vi "Autonomous Independent.vi"   [LabVIEW 2015]
doc: "This VI is called when autonomous begins, and will automatically be terminated when autonomous ends. You can carry out timed or sensor driven robot movement independently without needing to return to the caller."
uses:
  <vilib>/Rock Robotics/WPI/Utilities/WPI_GetSetVariantRefNum.vi
  <vilib>/Rock Robotics/Network Tables/NT Read Number.vi
  <vilib>/Rock Robotics/Network Tables/NT Write Numeric Array.vi
panel:
  # "Be sure to right-click and choose Data Operations>>Make Current Value default if you want to save the array values with the VI"
types:
  T1 = typedef "WPI_JoystickDevRef.ctl" = cluster{"Device":T2}
  T2 = typedef "WPI_JoystickDeviceEnum.ctl" = enum16{"USB 0", "USB 1", "USB 2", "USB 3", "USB 4", "USB 5"}
  T3 = typedef "WPI_EncoderDevRef.ctl" = cluster{"DevStatus":errorcluster, "EncoderIndex":T4, "CounterIndex":T5, "DistancePerCount":dbl, "Decoding Type":T6}
  T4 = typedef "FPGA_EncoderIdx.ctl" = enum8{"Enc 0", "Enc 1", "Enc 2", "Enc 3", "Enc 4", "Enc 5", "Enc 6", "Enc 7", "Invalid"}
  T5 = typedef "FPGA_CounterCtrSystemIndex.ctl" = enum8{"Ctr 0", "Ctr 1", "Ctr 2", "Ctr 3", "Ctr 4", "Ctr 5", "Ctr 6", "Ctr 7", "Invalid"}
  T6 = typedef "WPI_EncoderType.ctl" = enum16{"1x", "2x", "4x"}
  T7 = typedef "WPI_MotorControlDeviceRef.ctl" = cluster{"DeviceStatus":errorcluster, "Type":T8, "PWM":cluster{"PWM Channel":T9, "DeadBand":T10}, "CAN":cluster{"Device Number":u8, "Control Mode":T11, "Semaphore":T12, "Max Vout":dbl, "TalonSRX Control Mode":T13}, "Invert":bool}
  T8 = typedef "WPI_MotorControlType.ctl" = enum16{"PWM", "CAN", "CANTalonSRX"}
  T9 = typedef "FPGA_DIOPWMChannel.ctl" = enum8{"PWM 0", "PWM 1", "PWM 2", "PWM 3", "PWM 4", "PWM 5", "PWM 6", "PWM 7", "PWM 8", "PWM 9", "PWM MXP 0", "PWM MXP 1", "PWM MXP 2", "PWM MXP 3", "PWM MXP 4", "PWM MXP 5", "PWM MXP 6", "PWM MXP 7", "PWM MXP 8", "PWM MXP 9", "Invalid"}
  T10 = typedef "WPI_PWMDeadband.ctl" = cluster{"Name":string, "maxPositivePwm":i32, "minPositivePwm":i32, "centerPwm":i32, "maxNegativePwm":i32, "minNegativePwm":i32, "angularRange":u16}
  T11 = typedef "WPI_CANJaguar_ControlMode.ctl" = enum8{"Percent VBus", "Current", "Speed", "Position", "Voltage"}
  T12 = typedef "Semaphore RefNum" = refnum<k1>
  T13 = typedef "WPI_CANTalonSRX_APIControlMode.ctl" = enum8{"Percent VBus", "Speed", "Position", "Slave", "Unchanged / Invalid", "Voltage Compensation", "Current", "Motion Profile"}
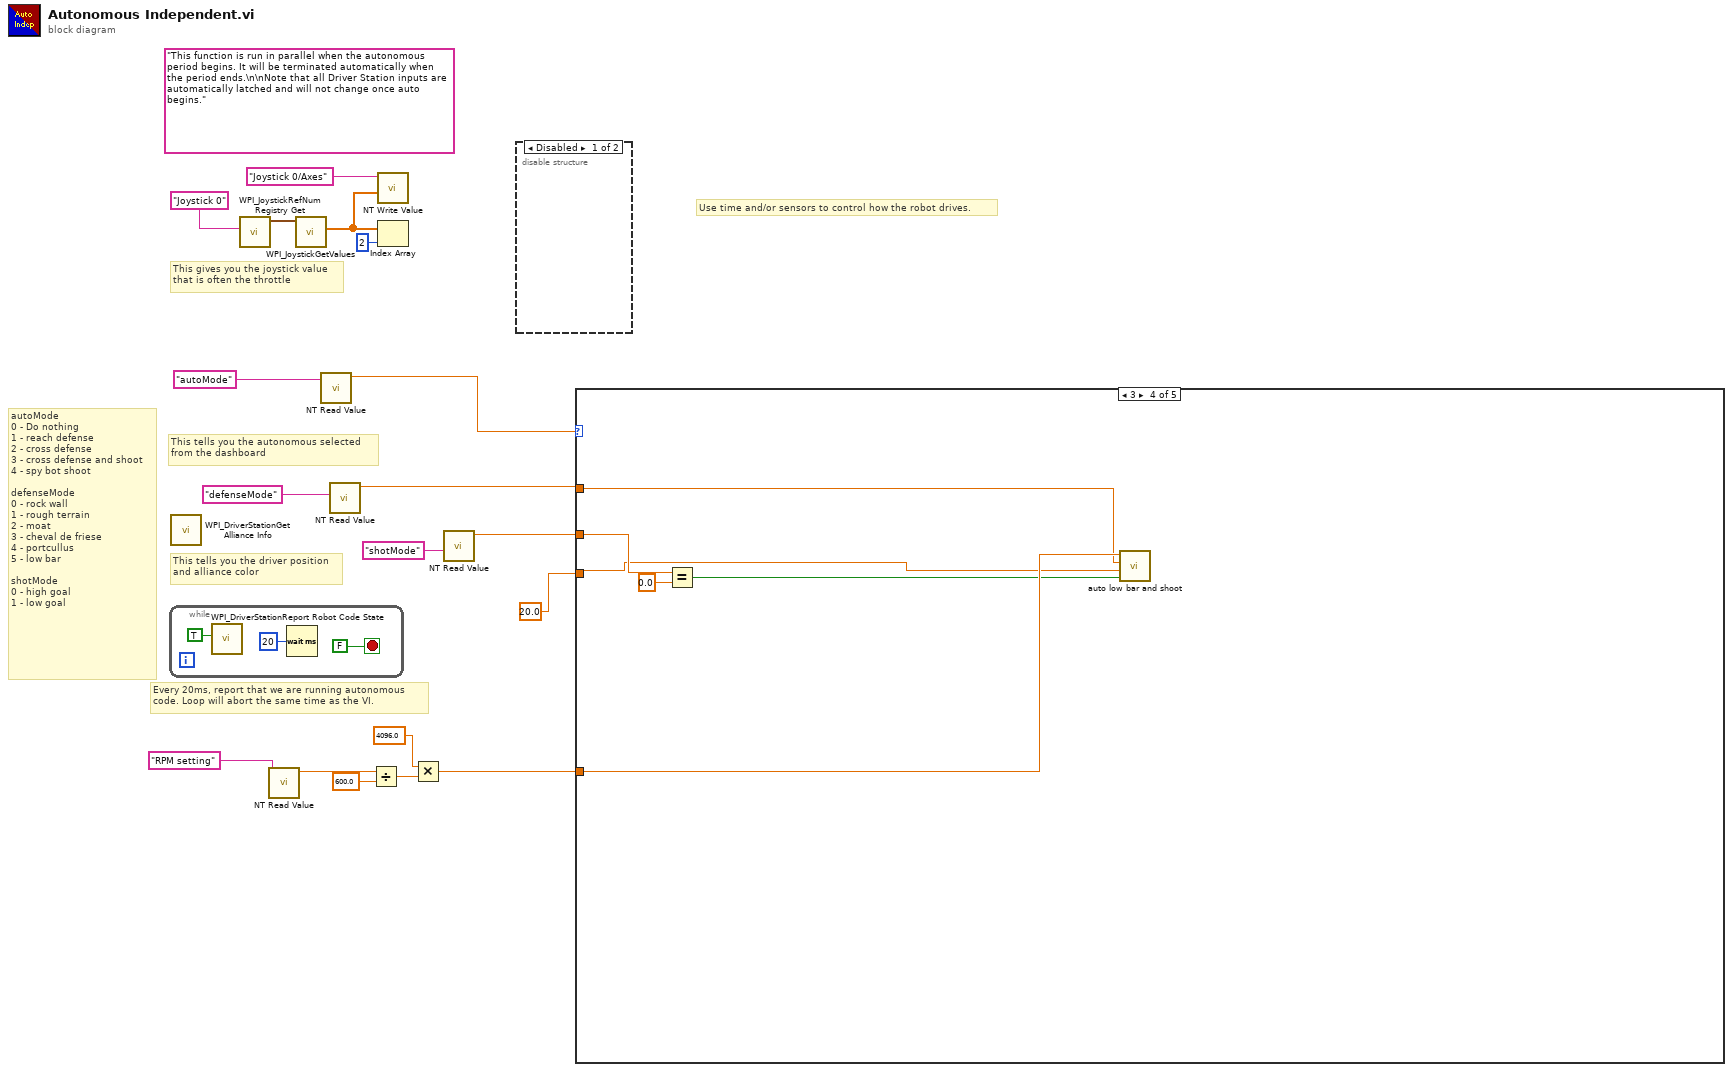
[diagram p0: block diagram]
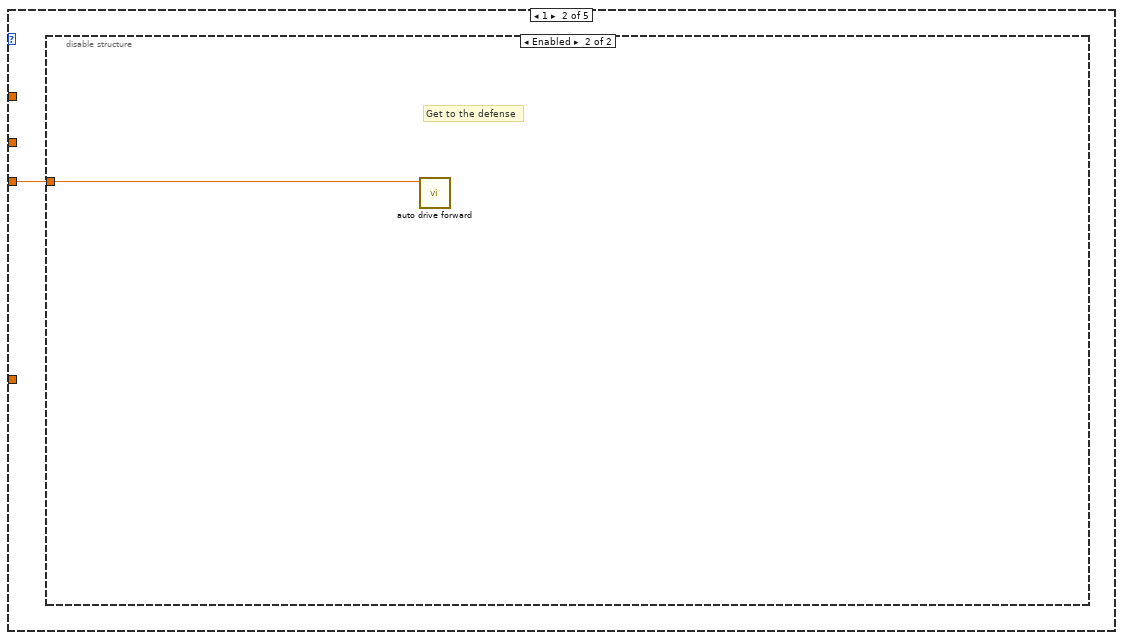
[diagram p3: hidden frame]
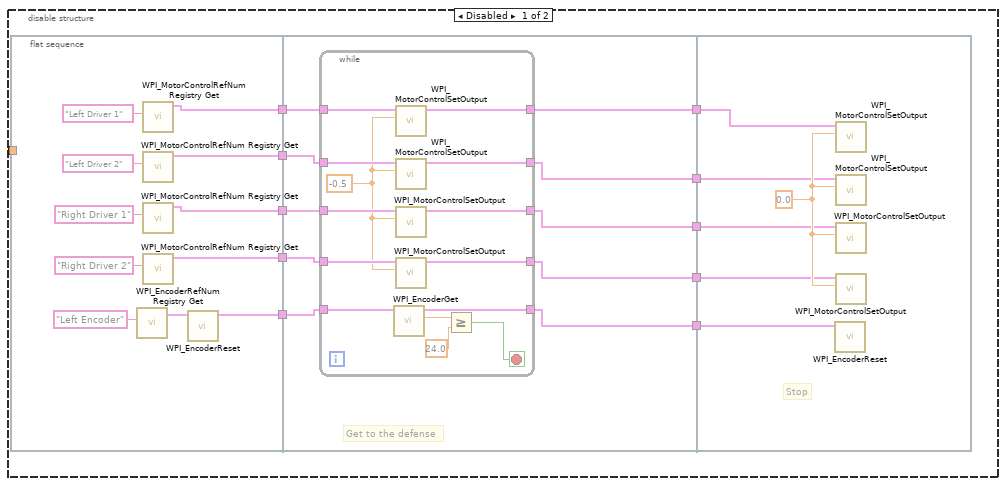
[diagram p4: hidden frame]
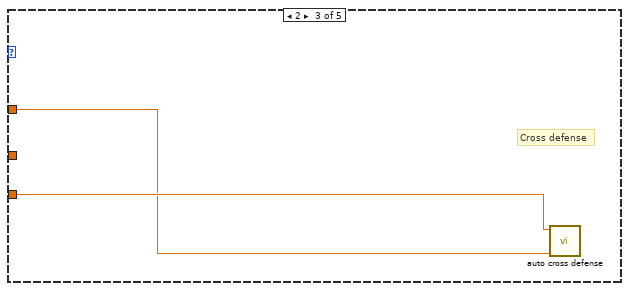
[diagram p5: hidden frame]
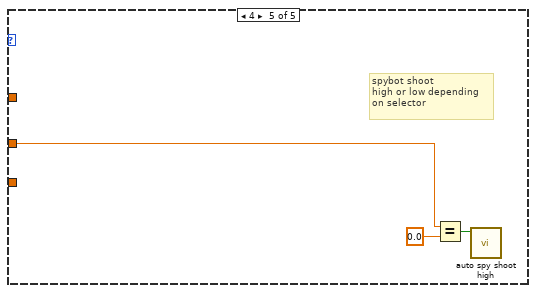
[diagram p6: hidden frame]
diagram:
  (unwired) "This function is run in parallel when the autonomous period begins. It will be terminated automatically when the period ends.\n\nNote that all Driver Station inputs are automatically latched and will not change once auto begins."
  # "autoMode\n0 - Do nothing\n1 - reach defense\n2 - cross defense\n3 - cross defense and shoot\n4 - spy bot shoot\n\ndefenseMode\n0 - rock wall\n1 - rough terrain\n2 - moat\n3 - cheval de friese\n4 - portcullus\n5 - low bar\n\nshotMode\n0 - high goal\n1 - low goal"
  # "This tells you the autonomous selected\nfrom the dashboard"
  # "Every 20ms, report that we are running autonomous\ncode. Loop will abort the same time as the VI."
  # "This gives you the joystick value\nthat is often the throttle"
  # "Use time and/or sensors to control how the robot drives."
  # "This tells you the driver position\nand alliance color"
  n1 = while {
    stop <- FALSE stop-if-true
    n2 = call <vilib>:"WPI_DriverStationReport Robot Code State.vi"("Autonomous"=TRUE) -> ()  [unwired: 10 in, 1 out]
    n3 = Wait (ms)(milliseconds to wait=u32 20) -> ()  [unwired: 1 out]
  }
  n4 = call <vilib>:"WPI_DriverStationGet Alliance Info.vi"() -> ()  [unwired: 12 out]
  n5 = call <vilib>:"WPI_JoystickRefNum Registry Get.vi"("refnum name"="Joystick 0") -> ("JoystickDevRef"=w17:T1)  [unwired: 1 in, 9 out]
  n6 = call-poly <vilib>:"NT Read Value.vi"("Name"="RPM setting") -> ("Numeric"=w5:dbl)  [unwired: 9 in, 1 out]
  n7 = call <vilib>:"WPI_JoystickGetValues.vi"("JoystickDevRef"=w17) -> ("Axes"=w14:dbl[])  [unwired: 6 in, 4 out]
  n8 = call-poly <vilib>:"NT Read Value.vi"("Name"="autoMode") -> ("Numeric"=w12:dbl)  [unwired: 9 in, 1 out]
  n9 = call-poly <vilib>:"NT Read Value.vi"("Name"="defenseMode") -> ("Numeric"=w9:dbl)  [unwired: 9 in, 1 out]
  n10 = Divide(x=w5, y=600.0) -> (x/y=w7:dbl)
  n11 = call-poly <vilib>:"NT Write Value.vi"("Numeric Array"=w14, "Name"="Joystick 0/Axes") -> ()  [unwired: 9 in, 1 out]
  n12 = Index Array(array=w14, index=2) -> ()  [unwired: 1 out]
  n13 = Multiply(x=4096.0, y=w7) -> (x*y=w6:dbl)
  n14 = call-poly <vilib>:"NT Read Value.vi"("Name"="shotMode") -> ("Numeric"=w1:dbl)  [unwired: 9 in, 1 out]
  n15 = disable-structure shown="Disabled" {
    frame Disabled {
    }
    frame Enabled {
    }
  }
  n16 = case shown="3" w12 {
    tunnel: 20.0 ("Distance") -> [_ w22 w76 w77 _]
    tunnel: w9 -> [_ _ w75 w78 _]
    tunnel: w6 -> [_ _ _ w82 _]
    tunnel: w1 -> [_ _ _ w81 w83]
    frame 0, Default {
      # "Do nothing"
    }
    frame 1 {
      n17 = disable-structure shown="Enabled" {
        disable-tunnel: w22 -> [_ w74]
        frame Disabled {
          n18 = flat-sequence {
            tunnel: [w33] -> w32
            tunnel: [w38] -> w31
            tunnel: [w37] -> w30
            tunnel: [w36] -> w29
            tunnel: [w35] -> w28
            tunnel: [w53] -> w27
            tunnel: [w52] -> w26
            tunnel: [w51] -> w25
            tunnel: [w50] -> w24
            tunnel: [w49] -> w23
            tunnel: w32 -> [w48]
            tunnel: w31 -> [w47]
            tunnel: w30 -> [w46]
            tunnel: w29 -> [w45]
            tunnel: w28 -> [w44]
            tunnel: w27 -> [w72]
            tunnel: w26 -> [w71]
            tunnel: w25 -> [w70]
            tunnel: w24 -> [w69]
            tunnel: w23 -> [w68]
            frame #0 {
              n19 = call <vilib>:"WPI_EncoderRefNum Registry Get.vi"("refnum name"="Left Encoder") -> ("EncoderDevRef"=w34:T3)  [unwired: 9 in, 1 out]
              n20 = call <vilib>:"WPI_MotorControlRefNum Registry Get.vi"("refnum name"="Left Driver 1") -> ("MotorControlDevRef"=w35:T7)  [unwired: 9 in, 1 out]
              n21 = call <vilib>:"WPI_MotorControlRefNum Registry Get.vi"("refnum name"="Left Driver 2") -> ("MotorControlDevRef"=w36:T7)  [unwired: 9 in, 1 out]
              n22 = call <vilib>:"WPI_MotorControlRefNum Registry Get.vi"("refnum name"="Right Driver 1") -> ("MotorControlDevRef"=w37:T7)  [unwired: 9 in, 1 out]
              n23 = call <vilib>:"WPI_MotorControlRefNum Registry Get.vi"("refnum name"="Right Driver 2") -> ("MotorControlDevRef"=w38:T7)  [unwired: 9 in, 1 out]
              n24 = call <vilib>:"WPI_EncoderReset.vi"("EncoderDevRef"=w34) -> ("EncoderDevRef"=w33:T3)  [unwired: 9 in, 1 out]
            }
            frame #1 {
              # "Get to the defense"
              n25 = while {
                tunnel: w44 -> [w67]
                tunnel: w45 -> [w66]
                tunnel: w46 -> [w65]
                tunnel: w47 -> [w64]
                tunnel: w48 -> [w62]
                tunnel: [w58] -> w53
                tunnel: [w57] -> w52
                tunnel: [w56] -> w51
                tunnel: [w55] -> w50
                tunnel: [w54] -> w49
                stop <- w60 stop-if-true
                w63 = -0.5 ("Output")
                n26 = call <vilib>:"WPI_EncoderGet.vi"("EncoderDevRef"=w62) -> ("Distance"=w61:dbl, "EncoderDevRef"=w54:T3)  [unwired: 5 in, 4 out]
                n27 = call <vilib>:"WPI_MotorControlSetOutput.vi"("Output"=w63, "MotorControlDevRef"=w67) -> ("MotorControlDevRef"=w58:T7)  [unwired: 7 in, 2 out]
                n28 = call <vilib>:"WPI_MotorControlSetOutput.vi"("Output"=w63, "MotorControlDevRef"=w66) -> ("MotorControlDevRef"=w57:T7)  [unwired: 7 in, 2 out]
                n29 = call <vilib>:"WPI_MotorControlSetOutput.vi"("Output"=w63, "MotorControlDevRef"=w65) -> ("MotorControlDevRef"=w56:T7)  [unwired: 7 in, 2 out]
                n30 = call <vilib>:"WPI_MotorControlSetOutput.vi"("Output"=w63, "MotorControlDevRef"=w64) -> ("MotorControlDevRef"=w55:T7)  [unwired: 7 in, 2 out]
                n31 = Greater Or Equal?(x=w61, y=24.0) -> (x >= y?=w60:bool)
              }
            }
            frame #2 {
              w73 = 0.0 ("Output")
              # "Stop"
              n32 = call <vilib>:"WPI_EncoderReset.vi"("EncoderDevRef"=w68) -> ()  [unwired: 9 in, 2 out]
              n33 = call <vilib>:"WPI_MotorControlSetOutput.vi"("Output"=w73, "MotorControlDevRef"=w72) -> ()  [unwired: 7 in, 3 out]
              n34 = call <vilib>:"WPI_MotorControlSetOutput.vi"("Output"=w73, "MotorControlDevRef"=w71) -> ()  [unwired: 7 in, 3 out]
              n35 = call <vilib>:"WPI_MotorControlSetOutput.vi"("Output"=w73, "MotorControlDevRef"=w70) -> ()  [unwired: 7 in, 3 out]
              n36 = call <vilib>:"WPI_MotorControlSetOutput.vi"("Output"=w73, "MotorControlDevRef"=w69) -> ()  [unwired: 7 in, 3 out]
            }
          }
        }
        frame Enabled {
          # "Get to the defense"
          n37 = call "auto drive forward.vi"("Distance"=w74) -> ()  [unwired: 11 in]
        }
      }
    }
    frame 2 {
      # "Cross defense"
      n38 = call "auto cross defense.vi"("Defense type"=w75, "Distance"=w76) -> ()  [unwired: 10 in]
    }
    frame 3 {
      n39 = Equal?(x=w81, y=0.0) -> (x = y?=w79:bool)
      n40 = call "auto low bar and shoot.vi"("high?"=w79, "Distance"=w77, "defenseMode"=w78, "RPM setting"=w82) -> ()  [unwired: 8 in]
    }
    frame 4 {
      # "spybot shoot \nhigh or low depending\non selector"
      n41 = Equal?(x=w83, y=0.0) -> (x = y?=w85:bool)
      n42 = call "auto spy shoot high.vi"("High?"=w85) -> ()  [unwired: 11 in]
    }
  }
